vi "arbwfm_loader.vi"(4 "Unit (0: Vpp)":u16(ring) items=["Vpp", "Vrms", "dB"], 5 "Frequency (1000 Hz)":dbl=1000.0 min=1e-06 max=80000000.0 format="%.2f", 7 "Offset (0.00 V)":dbl min=-10.0 max=10.0 format="%.2f", 9 "User Def. Wfm Name":string="WAVEFORM", 11 "VISA session":refnum<visa-resource-name>) -> (0 "error out":errorcluster)   [LabVIEW 2012]
doc: "Resets the instrument, uploads a waveform into its memory, configures the instrument to output uploaded waveform, and queries the instrument for user-defined waveforms currently loaded into its non-volatile memory."
uses:
  <vilib>/Utility/file.llb/Read From Spreadsheet File (DBL).vi
panel:
  in  "Amplitude (0.1 Vpp)":dbl=0.1 min=0.001 max=20.0 format="%.2f"
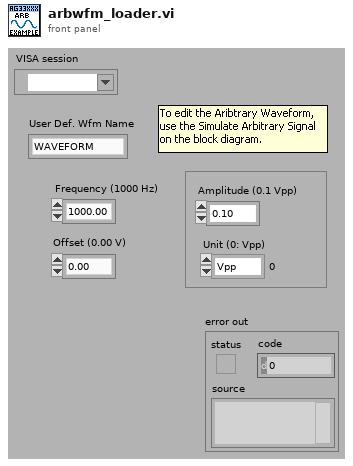
[diagram p1: front panel]
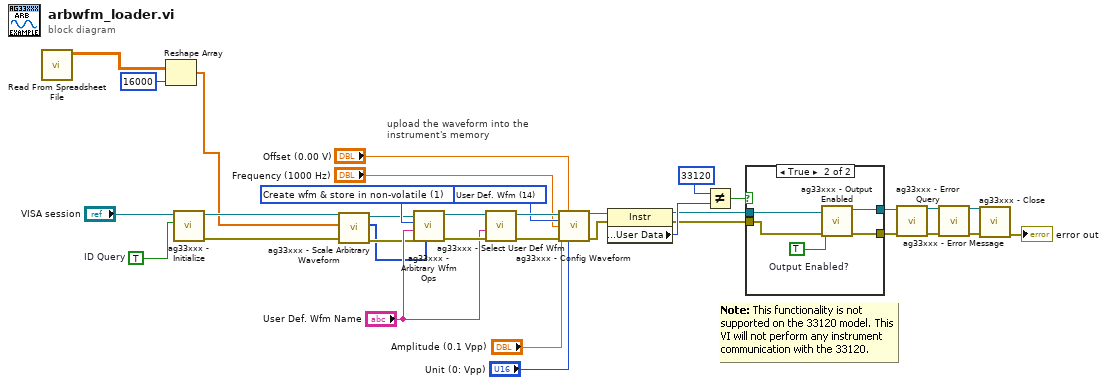
[diagram p0: block diagram]
diagram:
  w24 = TRUE  # ID Query
  w29 = u16 14 items=["DC"=0, "Sine"=1, "Square"=2, "Triangle"=3, "Ramp"=4, "Pulse"=6, "Noise"=7, "Sinc"=8, "Neg. Ramp"=9, "Exp. Rise"=10, "Exp. Fall"=11, "Cardiac"=12, "Volatile"=13, "User Def. Wfm"=14] ("Waveform Shape (1: Sine)")
  w31 = u16 1 items=["Create wfm & store in volatile", "Create wfm & store in non-volatile", "Copy wfm from volatile", "Delete wfm from volatile", "Delete one wfm from non-volatile", "Delete all wfms from non-volatile"] ("Mode (0: Create wfm & store in volatile)")
  # "upload the waveform into the instrument's memory"
  n1 = call-poly <vilib>:"Read From Spreadsheet File.vi"() -> ("all rows"=w3:dbl[][])  [unwired: 7 in, 4 out]
  n2 = Reshape Array(w3, 16000 ("dimension size")) -> (w1:dbl[])
  n3 = call <vilib>:"ag33xxx - Initialize.vi"("ID Query (T: Check)"=w24, "Instrument Resource Name"="VISA session") -> ("error out"=w22:errorcluster, "dup VISA session"=w23:refnum<visa-resource-name>)  [unwired: 8 in]
  n4 = call <vilib>:"ag33xxx - Scale Arbitrary Waveform.vi"("error in (no error)"=w22, "Data"=w1, "VISA resource name"=w23) -> ("error out"=w20:errorcluster, "Scaled Data"=w19:i16[], "VISA resource name out"=w21:refnum<visa-resource-name>)  [unwired: 6 in]
  n5 = call <vilib>:"ag33xxx - Arbitrary Wfm Ops.vi"("Data"=w19, "error in (no error)"=w20, "Waveform Name"="User Def. Wfm Name", "Mode (0: Create wfm & store in volatile)"=w31, "VISA session"=w21) -> ("error out"=w34:errorcluster, "dup VISA session"=w35:refnum<visa-resource-name>)  [unwired: 4 in, 1 out]
  n6 = call <vilib>:"ag33xxx - Select User Def Wfm.vi"("error in (no error)"=w34, "User Def. Wfm Name"="User Def. Wfm Name", "VISA session"=w35) -> ("error out"=w32:errorcluster, "dup VISA session"=w33:refnum<visa-resource-name>)  [unwired: 7 in]
  n7 = call <vilib>:"ag33xxx - Config Waveform.vi"("VISA session"=w33, "Offset (0.00 V)"="Offset (0.00 V)", "Waveform Shape (1: Sine)"=w29, "Frequency (1000 Hz)"="Frequency (1000 Hz)", "Amplitude (0.1 Vpp)"="Amplitude (0.1 Vpp)", "error in (no error)"=w32, "Unit (0: Vpp)"="Unit (0: Vpp)") -> ("dup VISA session"=w10:refnum<visa-resource-name>, "error out"=w9:errorcluster)  [unwired: 7 in]
  n8 = property class="Instr"(reference=w10, error in=w9) -> (reference out=w15:refnum<visa-resource-name>, error out=w14:errorcluster, "General Settings:User Data"=w18:u32)
  n9 = Not Equal?(x=u32 33120, y=w18) -> (x != y?=w16:bool)
  n10 = case shown="True" w16 {
    tunnel: w15 -> [w37 w41]
    tunnel: w14 -> [w36 w40]
    tunnel: [w37 w39] -> w12
    tunnel: [w36 w38] -> w13
    frame False {
    }
    frame True {
      w42 = TRUE  # Output Enabled?
      n11 = call <vilib>:"ag33xxx - Output Enabled.vi"("error in (no error)"=w40, "Output Enabled? (T: Yes)"=w42, "VISA session"=w41) -> ("error out"=w38:errorcluster, "dup VISA session"=w39:refnum<visa-resource-name>)  [unwired: 7 in]
    }
  }
  n12 = call <vilib>:"ag33xxx - Error Query.vi"("error in (no error)"=w13, "VISA session"=w12) -> ("error out"=w5:errorcluster, "dup VISA session"=w6:refnum<visa-resource-name>)  [unwired: 6 in, 2 out]
  n13 = call <vilib>:"ag33xxx - Error Message.vi"("VISA session"=w6, "error in (no error)"=w5) -> ("dup VISA session"=w8:refnum<visa-resource-name>, "error out"=w7:errorcluster)  [unwired: 9 in, 3 out]
  n14 = call <vilib>:"ag33xxx - Close.vi"("error in (no error)"=w7, "VISA session"=w8) -> ("error out"=→"error out":errorcluster)  [unwired: 9 in]
